vi "Denkovi Manager.vi"(7 "Action":T2=enum."Init", 8 "error in (no error)":errorcluster, 9 "Relay #":i8 min=1 max=8, 10 "Relays In":bool[](array[boolean])=[FALSE, FALSE, FALSE, FALSE, FALSE, FALSE, FALSE, FALSE, FALSE, FALSE, FALSE, FALSE, FALSE, FALSE, FALSE, FALSE]) -> (0 "error out":errorcluster, 2 "Relays Out":bool[](array[boolean]), 4 "Connected":bool)   [LabVIEW 2018]
uses:
  Denkovi Mngr.ctl
  <vilib>/Instr/_visa.llb/VISA Find Search Mode.ctl
  Hardware Globals.vi
panel:
  out "find list":string[](array[string])
  out "Device Description":string
  out "Pin States":T1
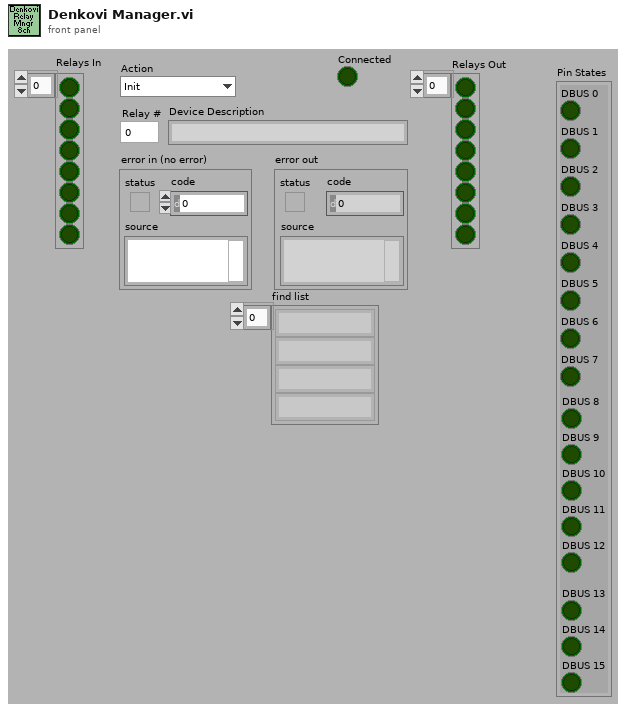
[diagram p1: front panel]
types:
  T1 = cluster{"DBUS 0":bool, "DBUS 1":bool, "DBUS 2":bool, "DBUS 3":bool, "DBUS 4":bool, "DBUS 5":bool, "DBUS 6":bool, "DBUS 7":bool, "DBUS 8":bool, "DBUS 9":bool, "DBUS 10":bool, "DBUS 11":bool, "DBUS 12":bool, "DBUS 13":bool, "DBUS 14":bool, "DBUS 15":bool}
  T2 = typedef "Denkovi Mngr.ctl" = enum16{"Search", "Init", "Set Peristaltic", "Set Vacuum", "Vac ON", "Vent&Close", "Set All Relays", "Set One Relay", "Read Relays", "Close"}
  T3 = typedef "VISA Find Search Mode.ctl" = u32
  T4 = cluster{"[0]":bool, "[1]":bool, "[2]":bool, "[3]":bool, "[4]":bool, "[5]":bool, "[6]":bool, "[7]":bool, "[8]":bool, "[9]":bool, "[10]":bool, "[11]":bool, "[12]":bool, "[13]":bool, "[14]":bool, "[15]":bool}
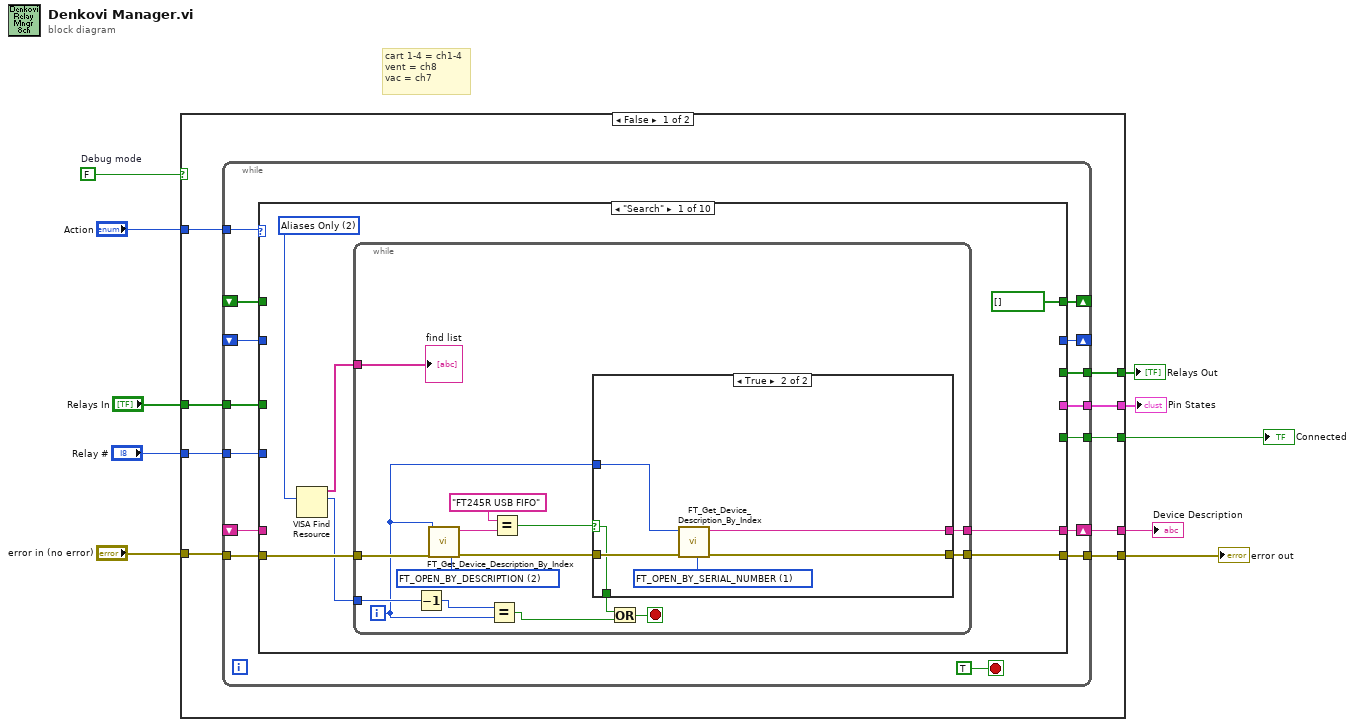
[diagram p0: block diagram]
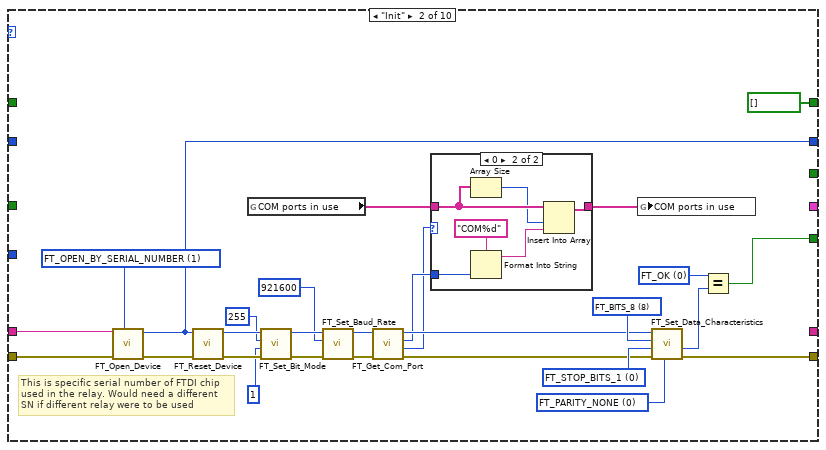
[diagram p3: hidden frame]
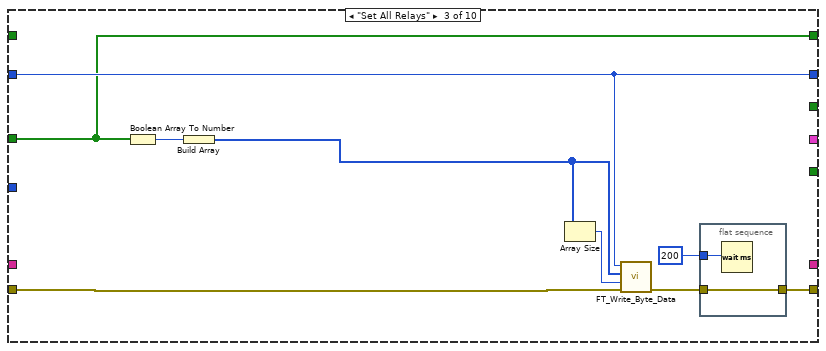
[diagram p5: hidden frame]
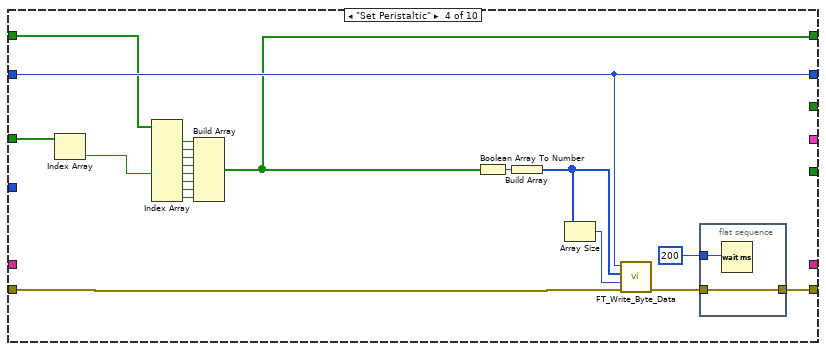
[diagram p6: hidden frame]
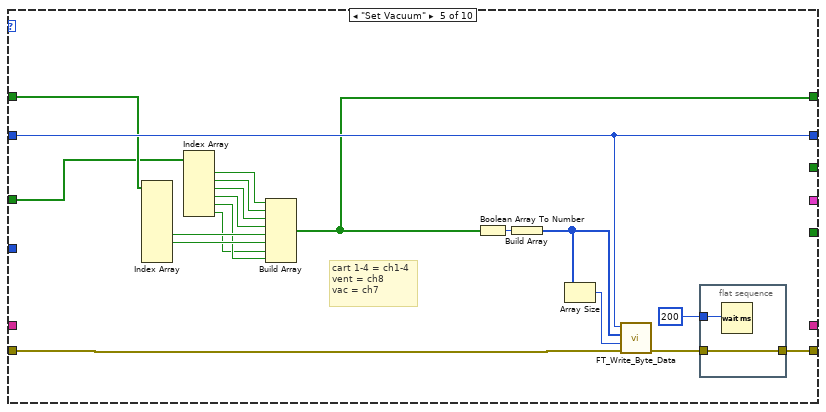
[diagram p7: hidden frame]
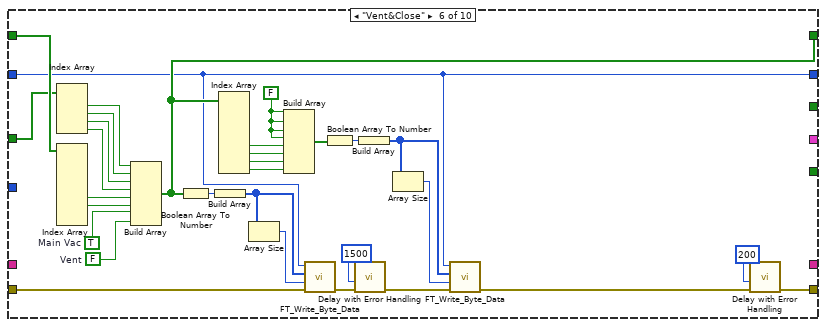
[diagram p8: hidden frame]
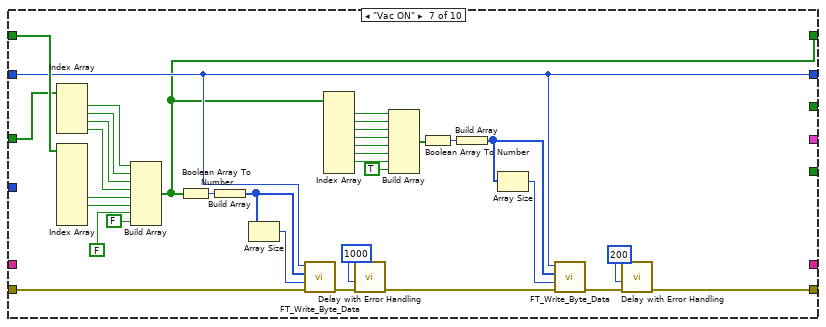
[diagram p9: hidden frame]
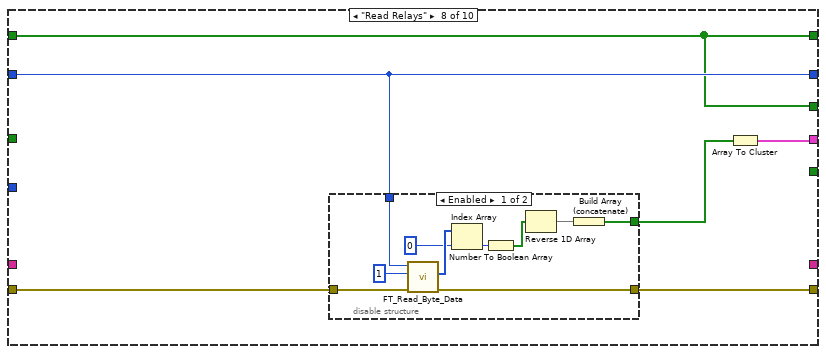
[diagram p10: hidden frame]
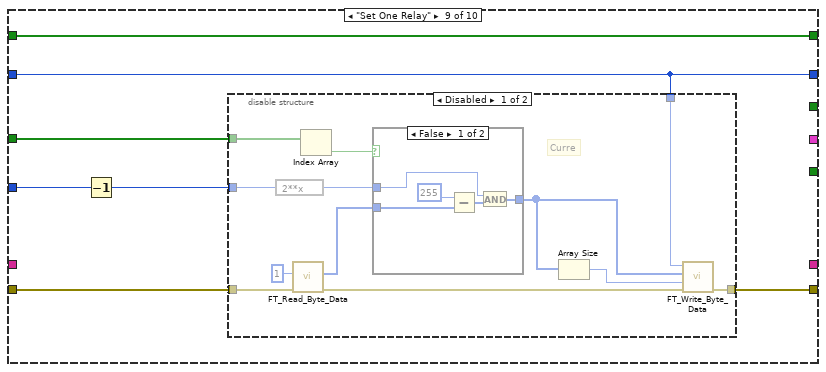
[diagram p12: hidden frame]
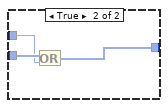
[diagram p13: hidden frame]
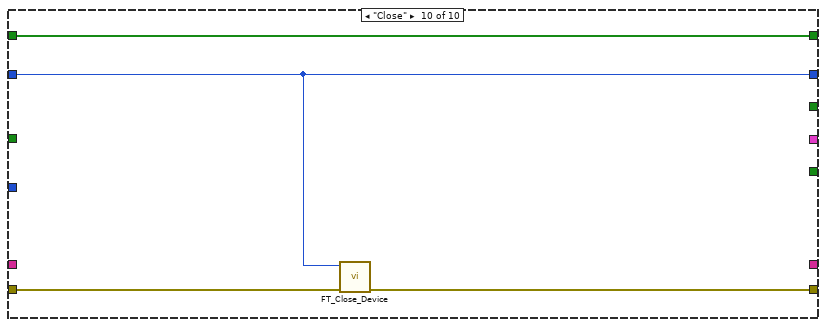
[diagram p15: hidden frame]
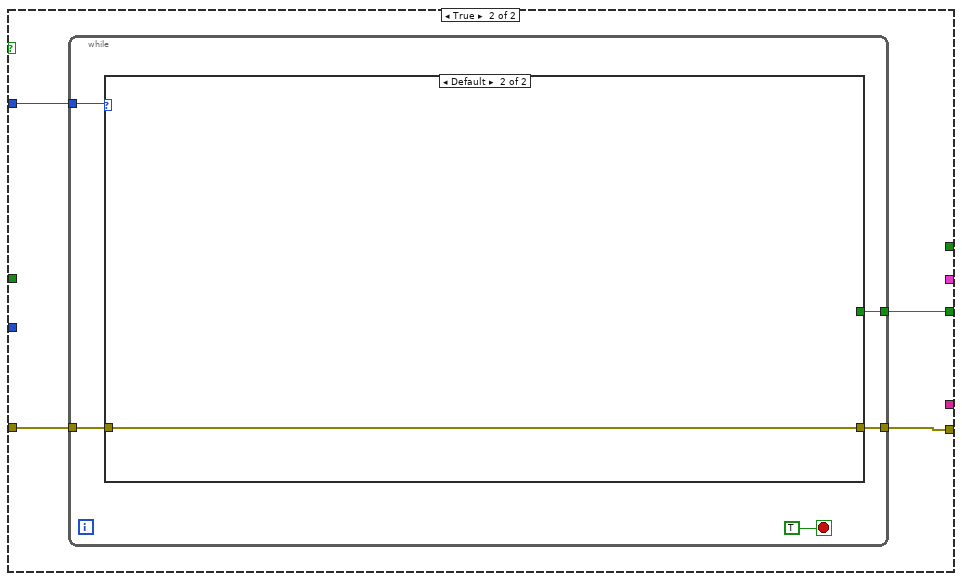
[diagram p16: hidden frame]
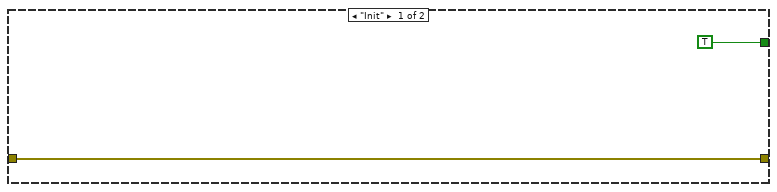
[diagram p17: hidden frame]
diagram:
  w2 = FALSE  # Debug mode
  # "cart 1-4 = ch1-4\nvent = ch8\nvac = ch7"
  n1 = case shown="False" w2 {
    tunnel: [w19 w268] -> w10
    tunnel: "error in (no error)" -> [w18 w267]
    tunnel: "Action" -> [w17 w266]
    tunnel: [w16 w265] -> w7
    tunnel: "Relays In" -> [w15 _]
    tunnel: [w14 _] -> w5
    tunnel: "Relay #" -> [w13 _]
    tunnel: [w12 _] -> w3
    tunnel: [w11 _] -> w1
    frame False {
      n2 = while {
        tunnel: w18 -> [w32]
        tunnel: [w31] -> w19
        tunnel: w17 -> [w33]
        tunnel: [w30] -> w16
        shift-right: [w29] -> _
        shift-left: _ -> [w28]
        tunnel: w15 -> [w27]
        tunnel: [w26] -> w14
        tunnel: w13 -> [w25]
        tunnel: [w24] -> w12
        shift-right: [w23] -> _
        shift-left: _ -> [w22]
        shift-right: [w21] -> w11
        shift-left: _ -> [w20]
        stop <- TRUE stop-if-true
        n3 = case shown="\"Search\"" w33 {
          tunnel: w32 -> [w41 w74 w101 w122 w143 w179 w213 w220 w236 w264]
          tunnel: [w38 w78 w103 w124 w145 w158 w200 w222 w239 w263] -> w31
          tunnel: [_ w91 _ _ _ _ _ _ _ _] -> w30
          tunnel: [_ w65 w105 w126 w147 w154 w192 w219 w238 w262] -> w29
          tunnel: w28 -> [_ _ w105 w126 w147 w154 w192 w219 w238 w262]
          tunnel: w27 -> [_ _ w99 w115 w138 w174 w208 _ w240 _]
          tunnel: [_ _ _ _ _ _ _ w221 _ _] -> w26
          tunnel: w25 -> [_ _ _ _ _ _ _ _ w237 _]
          tunnel: [_ _ _ _ _ _ _ w217 _ _] -> w24
          tunnel: [bool[] [] ("Relays In") bool[] [] ("Relays In") w99 w110 w133 w164 w185 w217 w234 w261] -> w23
          tunnel: w22 -> [_ _ _ w120 w141 w177 w211 w217 w234 w261]
          tunnel: [w35 _ _ _ _ _ _ _ _ _] -> w21
          tunnel: w20 -> [_ w64 _ _ _ _ _ _ _ _]
          frame "Search" {
            w40 = T3 2 items=["Canonical Names Only"=0, "Aliases Only"=2, "Include Matching Aliases"=3, "Include All Aliases"=4] ("Search Mode")
            n4 = VISA Find Resource(10:w40) -> (2:w39:u32, 3:w36:string[])  [unwired: 2 in, 1 out]
            n5 = while {
              tunnel: w41 -> [w56]
              tunnel: w39 -> [w51]
              tunnel: [w48] -> w38
              tunnel: w36 -> [w46]
              tunnel: [w45] -> w35
              i -> [w47]
              stop <- w44 stop-if-true
              w52 = u32 2 items=["FT_OPEN_BY_SERIAL_NUMBER"=1, "FT_OPEN_BY_DESCRIPTION"=2, "FT_OPEN_BY_LOCATION"=4] ("Flags")
              n6 = Decrement(x=w51) -> (x-1=w50:u32)
              n7 = call "FT_Get_Device_Description_By_Index.vi"("error in (no error)"=w56, "Flags"=w52, "Device Index"=w47) -> ("error out"=w53:errorcluster, "Device Description"=w55:string)  [unwired: 6 in, 1 out]
              n8 = Equal?(x=w50, y=w47) -> (x = y?=w43:bool)
              n9 = Equal?(x="FT245R USB FIFO", y=w55) -> (x = y?=w49:bool)
              n10 = case shown="True" w49 {
                selector: w49 -> [_ w58]
                tunnel: w53 -> [w57 w63]
                tunnel: [w57 w60] -> w48
                tunnel: w47 -> [_ w61]
                tunnel: [_ w59] -> w45
                tunnel: [_ w58] -> w42
                frame False {
                }
                frame True {
                  w62 = u32 1 items=["FT_OPEN_BY_SERIAL_NUMBER"=1, "FT_OPEN_BY_DESCRIPTION"=2, "FT_OPEN_BY_LOCATION"=4] ("Flags")
                  n11 = call "FT_Get_Device_Description_By_Index.vi"("error in (no error)"=w63, "Flags"=w62, "Device Index"=w61) -> ("error out"=w60:errorcluster, "Device Description"=w59:string)  [unwired: 6 in, 1 out]
                }
              }
              n12 = Or(x=w42, y=w43) -> (x .or. y?=w44:bool)
              "find list" <- w46
            }
          }
          frame "Init" {
            w75 = u32 1 items=["FT_OPEN_BY_SERIAL_NUMBER"=1, "FT_OPEN_BY_DESCRIPTION"=2, "FT_OPEN_BY_LOCATION"=4] ("Flags")
            w81 = u8 0 items=["FT_PARITY_NONE", "FT_PARITY_ODD", "FT_PARITY_EVEN", "FT_PARITY_MARK", "FT_PARITY_SPACE"] ("Parity")
            w82 = u8 0 items=["FT_STOP_BITS_1"=0, "FT_STOP_BITS_2"=2] ("Stop Bits")
            w80 = u8 8 items=["FT_BITS_7"=7, "FT_BITS_8"=8] ("Word Length")
            w90 = u32 0 items=["FT_OK", "FT_INVALID_HANDLE", "FT_DEVICE_NOT_FOUND", "FT_DEVICE_NOT_OPENED", "FT_IO_ERROR", "FT_INSUFFICIENT_RESOURCES", "FT_INVALID_PARAMETER", "FT_INVALID_BAUD_RATE", "FT_DEVICE_NOT_OPENED_FOR_ERASE", "FT_DEVICE_NOT_OPENED_FOR_WRITE", "FT_FAILED_TO_WRITE_DEVICE", "FT_EEPROM_READ_FAILED", "FT_EEPROM_WRITE_FAILED", "FT_EEPROM_ERASE_FAILED", "FT_EEPROM_NOT_PRESENT", "FT_EEPROM_NOT_PROGRAMMED", "FT_INVALID_ARGS", "FT_NOT_SUPPORTED", "FT_OTHER_ERROR"] ("FT_Status")
            # "This is specific serial number of FTDI chip\nused in the relay. Would need a different\nSN if different relay were to be used"
            n13 = call "FT_Open_Device.vi"("Flags"=w75, "error in (no error)"=w74, "Device Description"=w64) -> ("error out"=w77:errorcluster, "Handle"=w65:u64)  [unwired: 6 in, 1 out]
            n14 = call "FT_Reset_Device.vi"("error in (no error)"=w77, "Handle In"=w65) -> ("error out"=w89:errorcluster, "Handle Out"=w86:u64)  [unwired: 7 in, 1 out]
            n15 = global read "Hardware Globals.vi" "COM ports in use"() -> (w68:string[])
            n16 = call "FT_Set_Bit_Mode.vi"("error in (no error)"=w89, "Bit Mode"=u8 1 ("Bit Mode Mask"), "Bit Mode Mask"=u8 255, "Handle In"=w86) -> ("error out"=w88:errorcluster, "Handle Out"=w87:u64)  [unwired: 5 in, 1 out]
            n17 = call "FT_Set_Baud_Rate.vi"("error in (no error)"=w88, "Baud Rate"=921600, "Handle  In"=w87) -> ("error out"=w73:errorcluster, "Handle Out"=w72:u64)  [unwired: 6 in, 1 out]
            n18 = call "FT_Get_Com_Port.vi"("error in (no error)"=w73, "Handle In"=w72) -> ("error out"=w70:errorcluster, "FT_Status"=w66:u32, "ComPortNumber"=w69:i32, "Handle Out"=w71:u64)  [unwired: 6 in]
            n19 = case shown="0" w66 {
              tunnel: w69 -> [_ w98]
              tunnel: w68 -> [w92 w96]
              tunnel: [w92 w93] -> w67
              frame Default {
              }
              frame 0 {
                n20 = Array Size(array=w96) -> (size(s)=w95:i32)
                n21 = Format Into String(format string="COM%d", w98) -> (resulting string=w94:string)  [unwired: 2 in, 1 out]
                n22 = Insert Into Array(array=w96, index=w95, new element=w94) -> (w93:string[])
              }
            }
            n23 = global write "Hardware Globals.vi" "COM ports in use"(w67) -> ()
            n24 = call "FT_Set_Data_Characteristics.vi"("Parity"=w81, "error in"=w70, "Stop Bits"=w82, "Word Length"=w80, "Handle In"=w71) -> ("error out"=w78:errorcluster, "FT_Status"=w79:u32)  [unwired: 4 in, 1 out]
            n25 = Equal?(x=w90, y=w79) -> (x = y?=w91:bool)
          }
          frame "Set All Relays" {
            n26 = Boolean Array To Number(Boolean array=w99) -> (number=w100:u32)
            n27 = Build Array(w100) -> (w106:u32[])
            n28 = Array Size(array=w106) -> (size(s)=w107:i32)
            n29 = call "FT_Write_Byte_Data.vi"("error in (no error)"=w101, "Bytes To Write"=w107, "Buffer"=w106, "Handle"=w105) -> ("error out"=w104:errorcluster)  [unwired: 4 in, 3 out]
            n30 = flat-sequence {
              tunnel: w104 -> [w109]
              tunnel: [w109] -> w103
              tunnel: u32 200 ("Delay (ms)") -> [w108]
              frame #0 {
                n31 = Wait (ms)(milliseconds to wait=w108) -> ()  [unwired: 1 out]
              }
            }
          }
          frame "Set Peristaltic" {
            n32 = Index Array(array=w115) -> (element=w114:bool)  [unwired: 1 in]
            n33 = Index Array(array=w120) -> (element #1=w119:bool, element #2=w118:bool, element #3=w117:bool, element #4=w116:bool, element #6=w111:bool, element #7=w112:bool, element #8=w113:bool)  [unwired: 8 in, 1 out]
            n34 = Build Array(w119, w118, w117, w116, w114, w111, w112, w113) -> (w110:bool[])
            n35 = Boolean Array To Number(Boolean array=w110) -> (number=w121:u32)
            n36 = Build Array(w121) -> (w127:u32[])
            n37 = Array Size(array=w127) -> (size(s)=w128:i32)
            n38 = call "FT_Write_Byte_Data.vi"("error in (no error)"=w122, "Bytes To Write"=w128, "Buffer"=w127, "Handle"=w126) -> ("error out"=w125:errorcluster)  [unwired: 4 in, 3 out]
            n39 = flat-sequence {
              tunnel: w125 -> [w130]
              tunnel: [w130] -> w124
              tunnel: u32 200 ("Delay (ms)") -> [w129]
              frame #0 {
                n40 = Wait (ms)(milliseconds to wait=w129) -> ()  [unwired: 1 out]
              }
            }
          }
          frame "Set Vacuum" {
            # "cart 1-4 = ch1-4\nvent = ch8\nvac = ch7"
            n41 = Index Array(array=w141) -> (element #5=w139:bool, element #6=w140:bool)  [unwired: 8 in, 6 out]
            n42 = Index Array(array=w138) -> (element #1=w137:bool, element #2=w136:bool, element #3=w135:bool, element #4=w134:bool, element #5=w132:bool, element #6=w131:bool)  [unwired: 6 in]
            n43 = Build Array(w137, w136, w135, w134, w139, w140, w131, w132) -> (w133:bool[])
            n44 = Boolean Array To Number(Boolean array=w133) -> (number=w142:u32)
            n45 = Build Array(w142) -> (w148:u32[])
            n46 = Array Size(array=w148) -> (size(s)=w149:i32)
            n47 = call "FT_Write_Byte_Data.vi"("error in (no error)"=w143, "Bytes To Write"=w149, "Buffer"=w148, "Handle"=w147) -> ("error out"=w146:errorcluster)  [unwired: 4 in, 3 out]
            n48 = flat-sequence {
              tunnel: w146 -> [w151]
              tunnel: [w151] -> w145
              tunnel: u32 200 ("Delay (ms)") -> [w150]
              frame #0 {
                n49 = Wait (ms)(milliseconds to wait=w150) -> ()  [unwired: 1 out]
              }
            }
          }
          frame "Vent&Close" {
            w153 = TRUE  # Main Vac
            w160 = FALSE ("element")
            w169 = FALSE  # Vent
            n50 = Index Array(array=w174) -> (element #1=w173:bool, element #2=w172:bool, element #3=w171:bool, element #4=w170:bool)  [unwired: 4 in]
            n51 = Index Array(array=w177) -> (element #5=w175:bool, element #6=w176:bool)  [unwired: 8 in, 6 out]
            n52 = Build Array(w173, w172, w171, w170, w175, w176, w153, w169) -> (w164:bool[])
            n53 = Boolean Array To Number(Boolean array=w164) -> (number=w178:u32)
            n54 = Build Array(w178) -> (w181:u32[])
            n55 = Index Array(array=w164) -> (element #5=w163:bool, element #6=w162:bool, element #7=w161:bool, element #8=w156:bool)  [unwired: 8 in, 4 out]
            n56 = Array Size(array=w181) -> (size(s)=w182:i32)
            n57 = Build Array(w160, w160, w160, w160, w163, w162, w161, w156) -> (w155:bool[])
            n58 = call "FT_Write_Byte_Data.vi"("error in (no error)"=w179, "Bytes To Write"=w182, "Buffer"=w181, "Handle"=w154) -> ("error out"=w180:errorcluster)  [unwired: 4 in, 3 out]
            n59 = Boolean Array To Number(Boolean array=w155) -> (number=w167:u32)
            n60 = call "Delay with Error Handling.vi"("error in (no error)"=w180, "Delay (ms)"=u32 1500) -> ("error out"=w157:errorcluster)  [unwired: 9 in]
            n61 = Build Array(w167) -> (w166:u32[])
            n62 = Array Size(array=w166) -> (size(s)=w165:i32)
            n63 = call "FT_Write_Byte_Data.vi"("error in (no error)"=w157, "Bytes To Write"=w165, "Buffer"=w166, "Handle"=w154) -> ("error out"=w152:errorcluster)  [unwired: 4 in, 3 out]
            n64 = call "Delay with Error Handling.vi"("error in (no error)"=w152, "Delay (ms)"=u32 200) -> ("error out"=w158:errorcluster)  [unwired: 9 in]
          }
          frame "Vac ON" {
            n65 = Index Array(array=w208) -> (element #1=w207:bool, element #2=w206:bool, element #3=w205:bool, element #4=w204:bool)  [unwired: 4 in]
            n66 = Index Array(array=w211) -> (element #5=w209:bool, element #6=w210:bool)  [unwired: 8 in, 6 out]
            n67 = Build Array(w207, w206, w205, w204, w209, w210, FALSE ("element"), FALSE ("element")) -> (w185:bool[])
            n68 = Boolean Array To Number(Boolean array=w185) -> (number=w212:u32)
            n69 = Build Array(w212) -> (w215:u32[])
            n70 = Array Size(array=w215) -> (size(s)=w216:i32)
            n71 = call "FT_Write_Byte_Data.vi"("error in (no error)"=w213, "Bytes To Write"=w216, "Buffer"=w215, "Handle"=w192) -> ("error out"=w214:errorcluster)  [unwired: 4 in, 3 out]
            n72 = Index Array(array=w185) -> (element #1=w190:bool, element #2=w189:bool, element #3=w188:bool, element #4=w187:bool, element #5=w193:bool, element #6=w197:bool, element #7=w198:bool)  [unwired: 8 in, 1 out]
            n73 = call "Delay with Error Handling.vi"("error in (no error)"=w214, "Delay (ms)"=u32 1000) -> ("error out"=w184:errorcluster)  [unwired: 9 in]
            n74 = Build Array(w190, w189, w188, w187, w193, w197, w198, TRUE ("element")) -> (w199:bool[])
            n75 = Boolean Array To Number(Boolean array=w199) -> (number=w195:u32)
            n76 = Build Array(w195) -> (w191:u32[])
            n77 = Array Size(array=w191) -> (size(s)=w196:i32)
            n78 = call "FT_Write_Byte_Data.vi"("error in (no error)"=w184, "Bytes To Write"=w196, "Buffer"=w191, "Handle"=w192) -> ("error out"=w194:errorcluster)  [unwired: 4 in, 3 out]
            n79 = call "Delay with Error Handling.vi"("error in (no error)"=w194, "Delay (ms)"=u32 200) -> ("error out"=w200:errorcluster)  [unwired: 9 in]
          }
          frame "Read Relays" {
            n80 = disable-structure shown="Enabled" {
              disable-tunnel: [w232 w233] -> w222
              disable-tunnel: w220 -> [w231 w233]
              disable-tunnel: w219 -> [w230 _]
              disable-tunnel: [w223 _] -> w218
              frame Enabled {
                n81 = call "FT_Read_Byte_Data.vi"("error in (no error)"=w231, "Bytes To Read"=1, "Handle In"=w230) -> ("error out"=w232:errorcluster, "Read Data"=w226:u8[])  [unwired: 4 in, 3 out]
                n82 = Index Array(array=w226, index=0) -> (element=w225:u8)
                n83 = Number To Boolean Array(number=w225) -> (Boolean array=w228:bool[])
                n84 = Reverse 1D Array(array=w228) -> (reversed array=w227:bool[])
                n85 = Build Array (concatenate)(w227) -> (w223:bool[])
              }
              frame Disabled {
              }
            }
            n86 = Array To Cluster(array=w218) -> (cluster=w221:T4)
          }
          frame "Set One Relay" {
            n87 = Decrement(x=w237) -> (x-1=w235:i8)
            n88 = disable-structure shown="Disabled" {
              disable-tunnel: w240 -> [w251 _]
              disable-tunnel: [w250 _] -> w239
              disable-tunnel: w238 -> [w249 _]
              disable-tunnel: w236 -> [w246 _]
              disable-tunnel: w235 -> [w245 _]
              frame Disabled {
                # "Curre"
                n89 = expression code="2**x"(w245) -> (w242:i8)
                n90 = call "FT_Read_Byte_Data.vi"("error in (no error)"=w246, "Bytes To Read"=u32 1) -> ("error out"=w247:errorcluster, "Read Data"=w243:u8[])  [unwired: 5 in, 3 out]
                n91 = Index Array(array=w251) -> (element=w241:bool)  [unwired: 1 in]
                n92 = case shown="False" w241 {
                  tunnel: [w255 w258] -> w248
                  tunnel: w243 -> [w254 w260]
                  tunnel: w242 -> [w253 w259]
                  frame False {
                    n93 = Subtract(x=255, y=w254) -> (x-y=w257:i32[])
                    n94 = And(x=w253, y=w257) -> (x .and. y?=w255:i32[])
                  }
                  frame True {
                    n95 = Or(x=w260, y=w259) -> (x .or. y?=w258:u8[])
                  }
                }
                n96 = Array Size(array=w248) -> (size(s)=w252:i32)
                n97 = call "FT_Write_Byte_Data.vi"("error in (no error)"=w247, "Bytes To Write"=w252, "Buffer"=w248, "Handle"=w249) -> ("error out"=w250:errorcluster)  [unwired: 4 in, 3 out]
              }
              frame Enabled {
              }
            }
          }
          frame "Close" {
            n98 = call "FT_Close_Device.vi"("error in (no error)"=w264, "Handle In"=w262) -> ("error out"=w263:errorcluster)  [unwired: 7 in, 2 out]
          }
        }
      }
    }
    frame True {
      n99 = while {
        tunnel: w267 -> [w271]
        tunnel: [w270] -> w268
        tunnel: w266 -> [w272]
        tunnel: [w269] -> w265
        stop <- TRUE stop-if-true
        n100 = case shown="Default" w272 {
          tunnel: w271 -> [w274 w276]
          tunnel: [w274 w276] -> w270
          tunnel: [TRUE _] -> w269
          frame "Init" {
          }
          frame Default {
          }
        }
      }
    }
  }
  "error out" <- w10
  "Connected" <- w7
  "Pin States" <- w5
  "Relays Out" <- w3
  "Device Description" <- w1
